vi "Inc_Dec Amplitude.vi"(11 "Amplitude":T1(ring)) -> (0 "Pulse 4":dbl[](array[numeric]), 1 "Pulse 3":dbl[](array[numeric]), 2 "Pulse 2":dbl[](array[numeric]), 3 "Pulse 1":dbl[](array[numeric]), 4 "Index4":dbl[](array[numeric]), 5 "Index2":dbl[](array[numeric]), 6 "Index3":dbl[](array[numeric]), 7 "Index1":dbl[](array[numeric]))   [LabVIEW 2010]
panel:
  # "Current limits [A]"
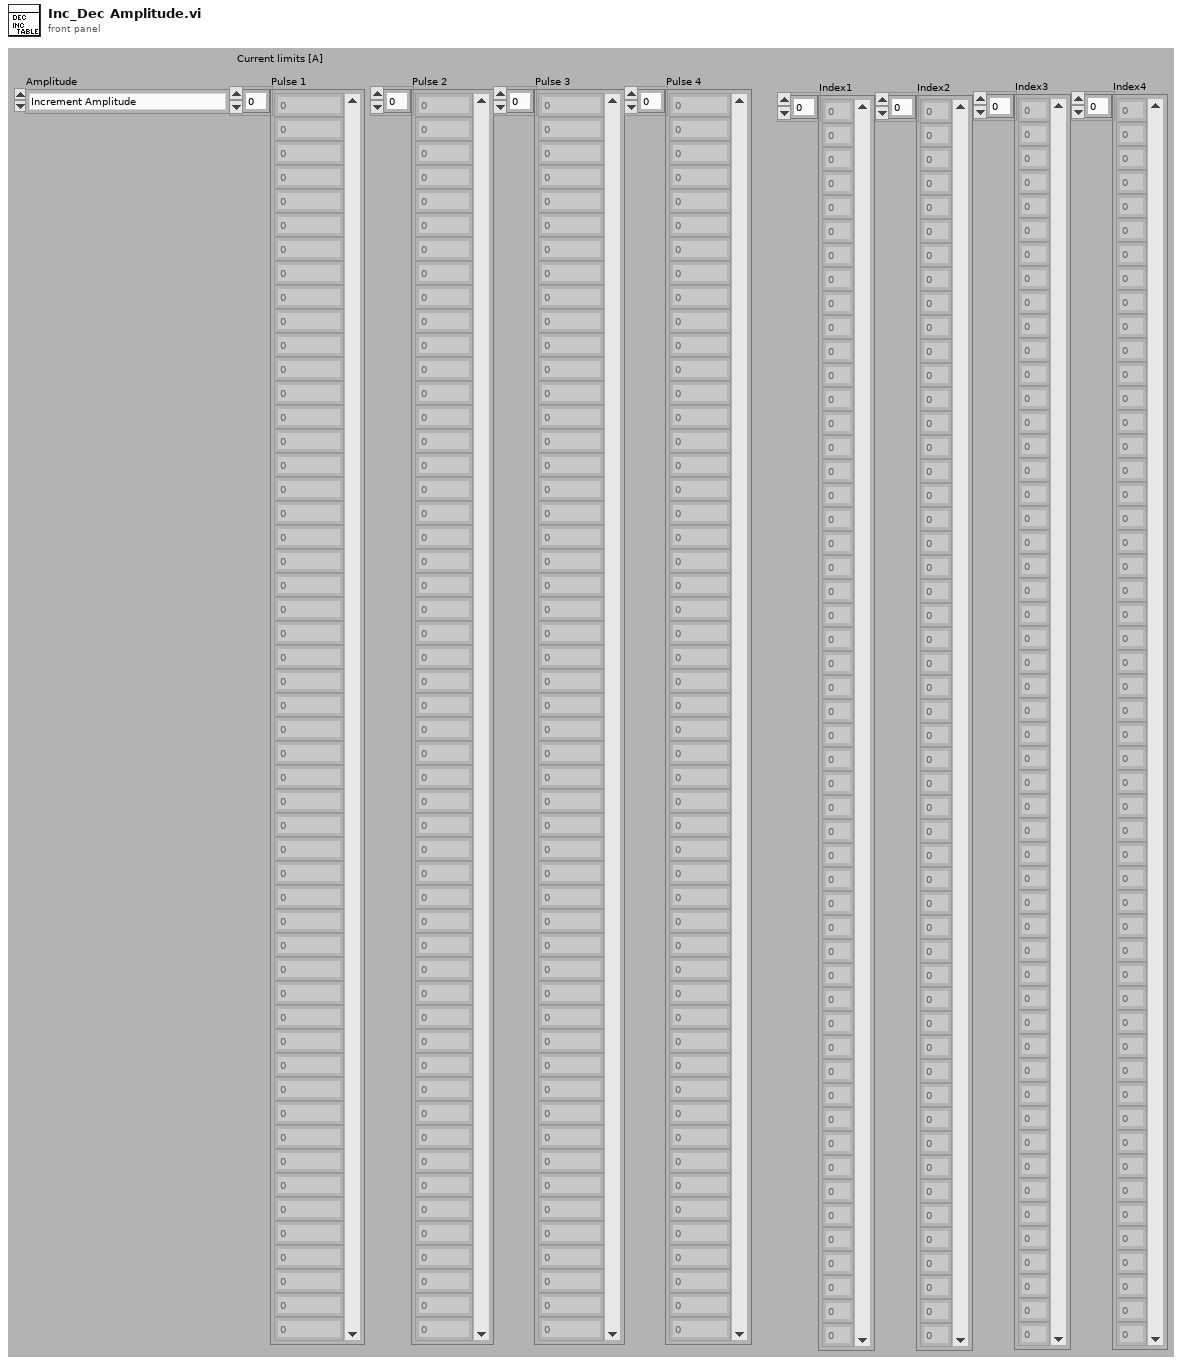
[diagram p1: front panel]
types:
  T1 = enum16{"Increment Amplitude", "Decrement Amplitude"}
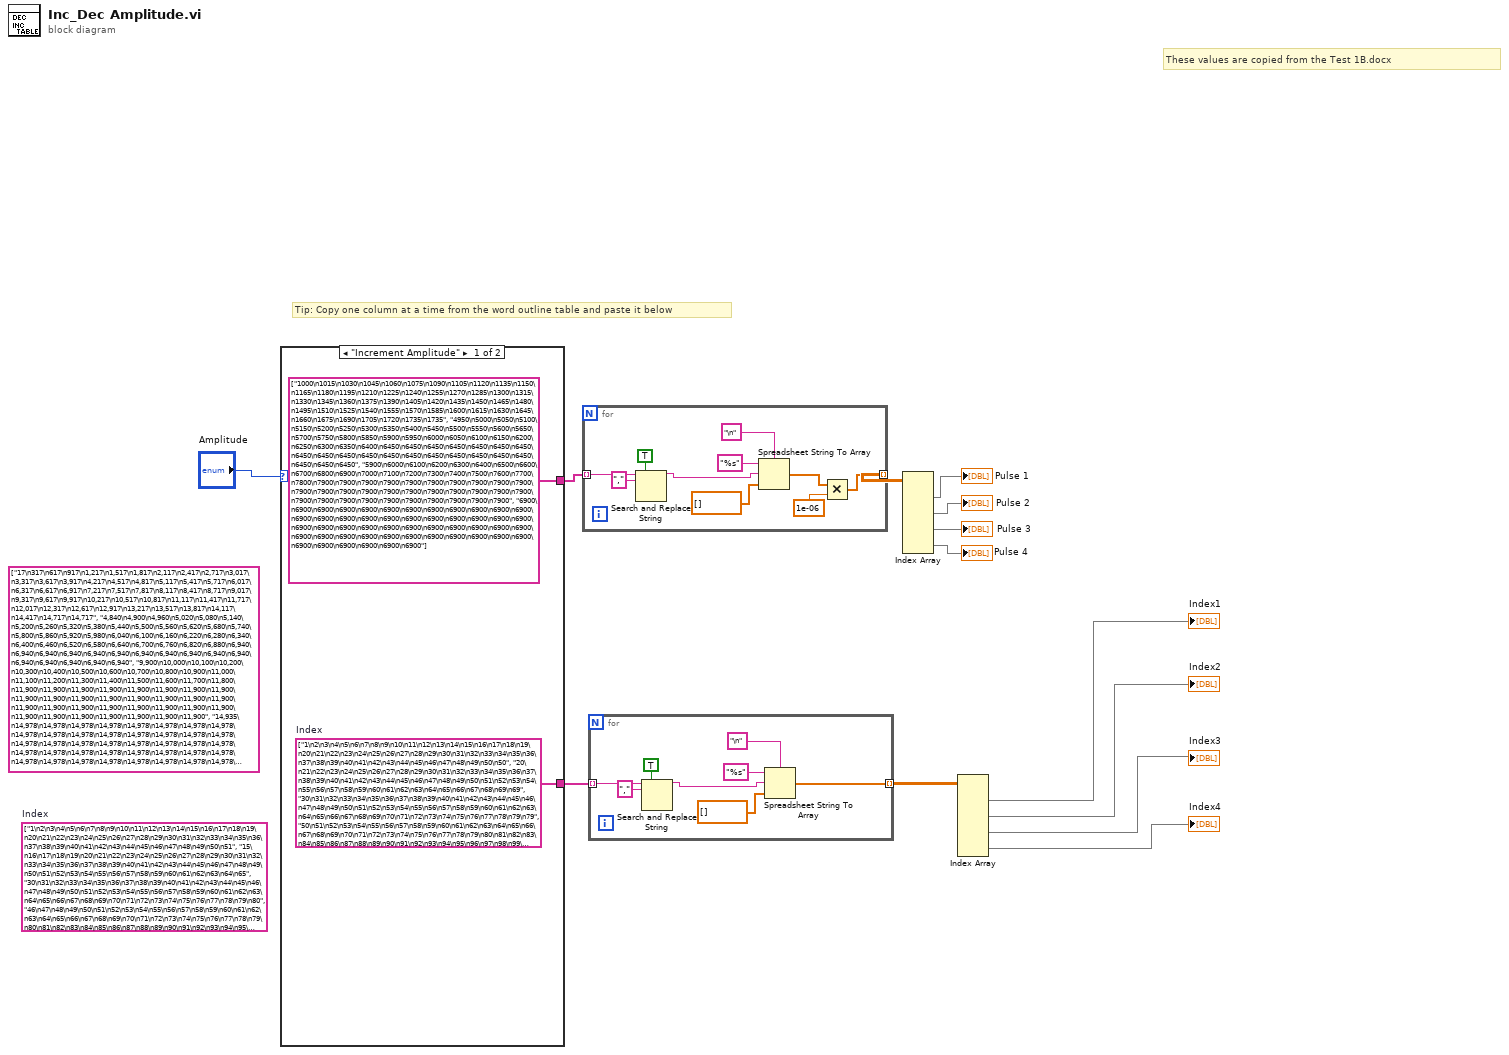
[diagram p0: block diagram]
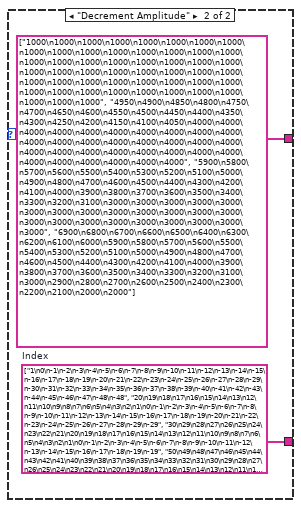
[diagram p2: hidden frame]
diagram:
  (unwired) string[] ["1\n2\n3\n4\n5\n6\n7\n8\n9\n10\n11\n12\n13\n14\n15\n16\n17\n18\n19\n20\n21\n22\n23\n24\n25\n26\n27\n28\n29\n30\n31\n32\n33\n34\n35\n36\n37\n38\n39\n40\n41\n42\n43\n44\n45\n46\n47\n48\n49\n50\n51", "15\n16\n17\n18\n19\n20\n21\n22\n23\n24\n25\n26\n27\n28\n29\n30\n31\n32\n33\n34\n35\n36\n37\n38\n39\n40\n41\n42\n43\n44\n45\n46\n47\n48\n49\n50\n51\n52\n53\n54\n55\n56\n57\n58\n59\n60\n61\n62\n63\n64\n65", "30\n31\n32\n33\n34\n35\n36\n37\n38\n39\n40\n41\n42\n43\n44\n45\n46\n47\n48\n49\n50\n51\n52\n53\n54\n55\n56\n57\n58\n59\n60\n61\n62\n63\n64\n65\n66\n67\n68\n69\n70\n71\n72\n73\n74\n75\n76\n77\n78\n79\n80", "46\n47\n48\n49\n50\n51\n52\n53\n54\n55\n56\n57\n58\n59\n60\n61\n62\n63\n64\n65\n66\n67\n68\n69\n70\n71\n72\n73\n74\n75\n76\n77\n78\n79\n80\n81\n82\n83\n84\n85\n86\n87\n88\n89\n90\n91\n92\n93\n94\n95\n96"]  # Index
  (unwired) string[] ["17\n317\n617\n917\n1,217\n1,517\n1,817\n2,117\n2,417\n2,717\n3,017\n3,317\n3,617\n3,917\n4,217\n4,517\n4,817\n5,117\n5,417\n5,717\n6,017\n6,317\n6,617\n6,917\n7,217\n7,517\n7,817\n8,117\n8,417\n8,717\n9,017\n9,317\n9,617\n9,917\n10,217\n10,517\n10,817\n11,117\n11,417\n11,717\n12,017\n12,317\n12,617\n12,917\n13,217\n13,517\n13,817\n14,117\n14,417\n14,717\n14,717", "4,840\n4,900\n4,960\n5,020\n5,080\n5,140\n5,200\n5,260\n5,320\n5,380\n5,440\n5,500\n5,560\n5,620\n5,680\n5,740\n5,800\n5,860\n5,920\n5,980\n6,040\n6,100\n6,160\n6,220\n6,280\n6,340\n6,400\n6,460\n6,520\n6,580\n6,640\n6,700\n6,760\n6,820\n6,880\n6,940\n6,940\n6,940\n6,940\n6,940\n6,940\n6,940\n6,940\n6,940\n6,940\n6,940\n6,940\n6,940\n6,940\n6,940\n6,940", "9,900\n10,000\n10,100\n10,200\n10,300\n10,400\n10,500\n10,600\n10,700\n10,800\n10,900\n11,000\n11,100\n11,200\n11,300\n11,400\n11,500\n11,600\n11,700\n11,800\n11,900\n11,900\n11,900\n11,900\n11,900\n11,900\n11,900\n11,900\n11,900\n11,900\n11,900\n11,900\n11,900\n11,900\n11,900\n11,900\n11,900\n11,900\n11,900\n11,900\n11,900\n11,900\n11,900\n11,900\n11,900\n11,900\n11,900\n11,900\n11,900\n11,900\n11,900", "14,935\n14,978\n14,978\n14,978\n14,978\n14,978\n14,978\n14,978\n14,978\n14,978\n14,978\n14,978\n14,978\n14,978\n14,978\n14,978\n14,978\n14,978\n14,978\n14,978\n14,978\n14,978\n14,978\n14,978\n14,978\n14,978\n14,978\n14,978\n14,978\n14,978\n14,978\n14,978\n14,978\n14,978\n14,978\n14,978\n14,978\n14,978\n14,978\n14,978\n14,978\n14,978\n14,978\n14,978\n14,978\n14,978\n14,978\n14,978\n14,978\n14,978\n14,978"]
  # "Tip: Copy one column at a time from the word outline table and paste it below"
  # "These values are copied from the Test 1B.docx"
  n1 = case shown="\"Increment Amplitude\"" "Amplitude" {
    tunnel: [string[] ["1000\n1015\n1030\n1045\n1060\n1075\n1090\n1105\n1120\n1135\n1150\n1165\n1180\n1195\n1210\n1225\n1240\n1255\n1270\n1285\n1300\n1315\n1330\n1345\n1360\n1375\n1390\n1405\n1420\n1435\n1450\n1465\n1480\n1495\n1510\n1525\n1540\n1555\n1570\n1585\n1600\n1615\n1630\n1645\n1660\n1675\n1690\n1705\n1720\n1735\n1735", "4950\n5000\n5050\n5100\n5150\n5200\n5250\n5300\n5350\n5400\n5450\n5500\n5550\n5600\n5650\n5700\n5750\n5800\n5850\n5900\n5950\n6000\n6050\n6100\n6150\n6200\n6250\n6300\n6350\n6400\n6450\n6450\n6450\n6450\n6450\n6450\n6450\n6450\n6450\n6450\n6450\n6450\n6450\n6450\n6450\n6450\n6450\n6450\n6450\n6450\n6450", "5900\n6000\n6100\n6200\n6300\n6400\n6500\n6600\n6700\n6800\n6900\n7000\n7100\n7200\n7300\n7400\n7500\n7600\n7700\n7800\n7900\n7900\n7900\n7900\n7900\n7900\n7900\n7900\n7900\n7900\n7900\n7900\n7900\n7900\n7900\n7900\n7900\n7900\n7900\n7900\n7900\n7900\n7900\n7900\n7900\n7900\n7900\n7900\n7900\n7900\n7900", "6900\n6900\n6900\n6900\n6900\n6900\n6900\n6900\n6900\n6900\n6900\n6900\n6900\n6900\n6900\n6900\n6900\n6900\n6900\n6900\n6900\n6900\n6900\n6900\n6900\n6900\n6900\n6900\n6900\n6900\n6900\n6900\n6900\n6900\n6900\n6900\n6900\n6900\n6900\n6900\n6900\n6900\n6900\n6900\n6900\n6900\n6900\n6900\n6900\n6900\n6900"] string[] ["1000\n1000\n1000\n1000\n1000\n1000\n1000\n1000\n1000\n1000\n1000\n1000\n1000\n1000\n1000\n1000\n1000\n1000\n1000\n1000\n1000\n1000\n1000\n1000\n1000\n1000\n1000\n1000\n1000\n1000\n1000\n1000\n1000\n1000\n1000\n1000\n1000\n1000\n1000\n1000\n1000\n1000\n1000\n1000\n1000\n1000\n1000\n1000\n1000\n1000\n1000", "4950\n4900\n4850\n4800\n4750\n4700\n4650\n4600\n4550\n4500\n4450\n4400\n4350\n4300\n4250\n4200\n4150\n4100\n4050\n4000\n4000\n4000\n4000\n4000\n4000\n4000\n4000\n4000\n4000\n4000\n4000\n4000\n4000\n4000\n4000\n4000\n4000\n4000\n4000\n4000\n4000\n4000\n4000\n4000\n4000\n4000\n4000\n4000\n4000\n4000\n4000", "5900\n5800\n5700\n5600\n5500\n5400\n5300\n5200\n5100\n5000\n4900\n4800\n4700\n4600\n4500\n4400\n4300\n4200\n4100\n4000\n3900\n3800\n3700\n3600\n3500\n3400\n3300\n3200\n3100\n3000\n3000\n3000\n3000\n3000\n3000\n3000\n3000\n3000\n3000\n3000\n3000\n3000\n3000\n3000\n3000\n3000\n3000\n3000\n3000\n3000\n3000", "6900\n6800\n6700\n6600\n6500\n6400\n6300\n6200\n6100\n6000\n5900\n5800\n5700\n5600\n5500\n5400\n5300\n5200\n5100\n5000\n4900\n4800\n4700\n4600\n4500\n4400\n4300\n4200\n4100\n4000\n3900\n3800\n3700\n3600\n3500\n3400\n3300\n3200\n3100\n3000\n2900\n2800\n2700\n2600\n2500\n2400\n2300\n2200\n2100\n2000\n2000"]] -> w13
    tunnel: [w14 w16] -> w1
    frame "Increment Amplitude" {
      w14 = string[] ["1\n2\n3\n4\n5\n6\n7\n8\n9\n10\n11\n12\n13\n14\n15\n16\n17\n18\n19\n20\n21\n22\n23\n24\n25\n26\n27\n28\n29\n30\n31\n32\n33\n34\n35\n36\n37\n38\n39\n40\n41\n42\n43\n44\n45\n46\n47\n48\n49\n50\n50", "20\n21\n22\n23\n24\n25\n26\n27\n28\n29\n30\n31\n32\n33\n34\n35\n36\n37\n38\n39\n40\n41\n42\n43\n44\n45\n46\n47\n48\n49\n50\n51\n52\n53\n54\n55\n56\n57\n58\n59\n60\n61\n62\n63\n64\n65\n66\n67\n68\n69\n69", "30\n31\n32\n33\n34\n35\n36\n37\n38\n39\n40\n41\n42\n43\n44\n45\n46\n47\n48\n49\n50\n51\n52\n53\n54\n55\n56\n57\n58\n59\n60\n61\n62\n63\n64\n65\n66\n67\n68\n69\n70\n71\n72\n73\n74\n75\n76\n77\n78\n79\n79", "50\n51\n52\n53\n54\n55\n56\n57\n58\n59\n60\n61\n62\n63\n64\n65\n66\n67\n68\n69\n70\n71\n72\n73\n74\n75\n76\n77\n78\n79\n80\n81\n82\n83\n84\n85\n86\n87\n88\n89\n90\n91\n92\n93\n94\n95\n96\n97\n98\n99\n99"]  # Index
    }
    frame "Decrement Amplitude" {
      w16 = string[] ["1\n0\n-1\n-2\n-3\n-4\n-5\n-6\n-7\n-8\n-9\n-10\n-11\n-12\n-13\n-14\n-15\n-16\n-17\n-18\n-19\n-20\n-21\n-22\n-23\n-24\n-25\n-26\n-27\n-28\n-29\n-30\n-31\n-32\n-33\n-34\n-35\n-36\n-37\n-38\n-39\n-40\n-41\n-42\n-43\n-44\n-45\n-46\n-47\n-48\n-48", "20\n19\n18\n17\n16\n15\n14\n13\n12\n11\n10\n9\n8\n7\n6\n5\n4\n3\n2\n1\n0\n-1\n-2\n-3\n-4\n-5\n-6\n-7\n-8\n-9\n-10\n-11\n-12\n-13\n-14\n-15\n-16\n-17\n-18\n-19\n-20\n-21\n-22\n-23\n-24\n-25\n-26\n-27\n-28\n-29\n-29", "30\n29\n28\n27\n26\n25\n24\n23\n22\n21\n20\n19\n18\n17\n16\n15\n14\n13\n12\n11\n10\n9\n8\n7\n6\n5\n4\n3\n2\n1\n0\n-1\n-2\n-3\n-4\n-5\n-6\n-7\n-8\n-9\n-10\n-11\n-12\n-13\n-14\n-15\n-16\n-17\n-18\n-19\n-19", "50\n49\n48\n47\n46\n45\n44\n43\n42\n41\n40\n39\n38\n37\n36\n35\n34\n33\n32\n31\n30\n29\n28\n27\n26\n25\n24\n23\n22\n21\n20\n19\n18\n17\n16\n15\n14\n13\n12\n11\n10\n9\n8\n7\n6\n5\n4\n3\n2\n1\n1"]  # Index
    }
  }
  n2 = for {
    tunnel: w13 -> [w24] mode=indexing
    tunnel: [w19] -> w12 mode=indexing
    n3 = Search and Replace String(replace all?=TRUE ("replace all? (F)"), input string=w24, search string=",") -> (result string=w23:string)  [unwired: 5 in, 3 out]
    n4 = Spreadsheet String To Array(delimiter (Tab)="\n", format string="%s", spreadsheet string=w23, array type (2D Dbl)=dbl[] []) -> (array=w20:dbl[])
    n5 = Multiply(x=w20, y=1e-06) -> (x*y=w19:dbl[])
  }
  n6 = for {
    tunnel: w1 -> [w32] mode=indexing
    tunnel: [w28] -> w6 mode=indexing
    n7 = Search and Replace String(replace all?=TRUE ("replace all? (F)"), input string=w32, search string=",") -> (result string=w31:string)  [unwired: 5 in, 3 out]
    n8 = Spreadsheet String To Array(delimiter (Tab)="\n", format string="%s", spreadsheet string=w31, array type (2D Dbl)=dbl[] []) -> (array=w28:dbl[])
  }
  n9 = Index Array(array=w12) -> (element #1=→"Pulse 1":dbl[], element #2=→"Pulse 2":dbl[], element #3=→"Pulse 3":dbl[], element #4=→"Pulse 4":dbl[])  [unwired: 8 in]
  n10 = Index Array(array=w6) -> (element #1=→"Index1":dbl[], element #2=→"Index2":dbl[], element #3=→"Index3":dbl[], element #4=→"Index4":dbl[])  [unwired: 8 in]
